vi "Multiple Zeroes.vi"(11 "p":dbl[](array[numeric])) -> (3 "sequence of polynomials":dbl[][](array[numeric]))   [LabVIEW 2014, in "NI_AALPro.lvlib"]
doc: "From ../labview/vi.lib/gmath/zeros.llb."
uses:
  NI_AALPro.lvlib
  Ramp Pattern by Samples.vi
  NI_AALBase.lvlib
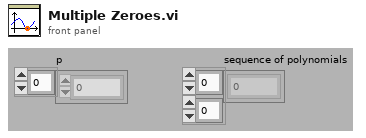
[diagram p1: front panel]
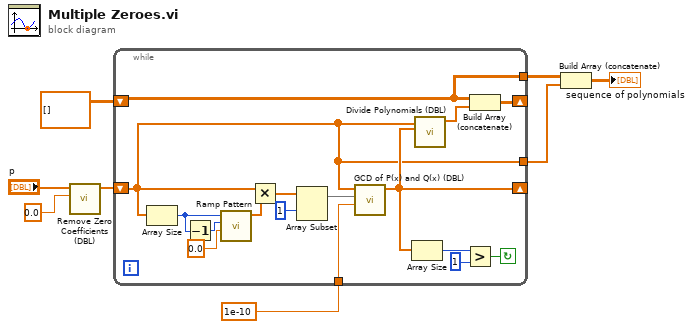
[diagram p0: block diagram]
diagram:
  n1 = call "Remove Zero Coefficients (DBL).vi"("threshold"=0.0, "P(x) In"="p") -> ("P(x) Out"=w5:dbl[])  [unwired: 7 in, 2 out]
  n2 = while {
    tunnel: [w11] -> w7
    tunnel: [w18] -> w8
    shift-left: w5 -> [w11]
    shift-right: [w17] -> _
    shift-left: dbl[][] [] -> [w18]
    shift-right: [w20] -> _
    tunnel: 1e-10 ("eps for GCD") -> [w15]
    stop <- w22 continue-if-true
    n3 = Array Size(array=w11) -> (size(s)=w14:i32)
    n4 = Decrement(x=w14) -> (x-1=w13:i32)
    n5 = call-poly "Ramp Pattern.vi"("start"=0.0, "end"=w13, "samples"=w14) -> ("Ramp Pattern"=w10:dbl[])  [unwired: 7 in, 1 out]
    n6 = Multiply(x=w11, y=w10) -> (x*y=w9:dbl[])
    n7 = Array Subset(array=w9, index=1) -> (w19:dbl[])  [unwired: 1 in]
    n8 = call "GCD of P(x) and Q(x) (DBL).vi"("tolerance"=w15, "Q(x)"=w19, "P(x)"=w11) -> ("Greatest Common Divisor"=w17:dbl[])  [unwired: 7 in, 1 out]
    n9 = Array Size(array=w17) -> (size(s)=w23:i32)
    n10 = call "Divide Polynomials (DBL).vi"("Q(x)"=w17, "P(x)"=w11) -> ("P(x)/Q(x)"=w16:dbl[])  [unwired: 7 in, 2 out]
    n11 = Greater?(x=w23, y=1) -> (0:w22:bool)
    n12 = Build Array (concatenate)(w18, w16) -> (w20:dbl[][])
  }
  n13 = Build Array (concatenate)(w8, w7) -> (→"sequence of polynomials":dbl[][])
